vi "Remove Lens Distortion.vi"(2 "error in (no error)":errorcluster, 3 "Image Dst":T1, 4 "Calibration Image":T1) -> (0 "error out":errorcluster, 1 "Corrected Image":T1)   [LabVIEW 2009, in "Camera.lvlib" / "Lens Distortion.lvlib"]
doc: "Removes lens distortion in a image using a calibration image"
uses:
  <vilib>/vision/Image Controls.llb/IMAQ Image.ctl
  Lens Distortion.lvlib
  <vilib>/vision/NI_Vision_Development_Module.lvlib
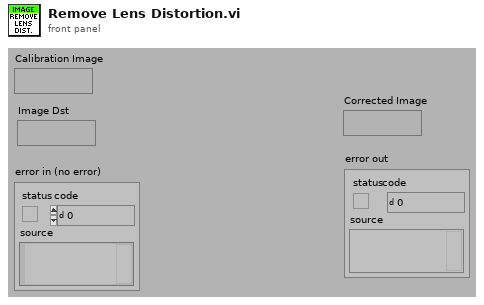
[diagram p1: front panel]
types:
  T1 = typedef "IMAQ Image.ctl" = refnum<image>
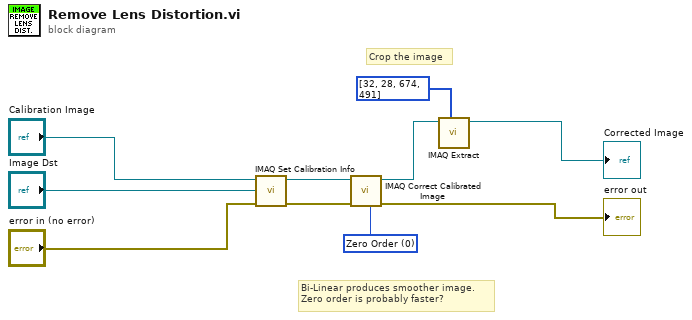
[diagram p0: block diagram]
diagram:
  w10 = u32 0 items=["Zero Order", "Bi-Linear", "Quadratic", "Cubic Spline"] ("Interpolation Type")
  # "Crop the image"
  # "Bi-Linear produces smoother image.\nZero order is probably faster?"
  n1 = call "IMAQ Set Calibration Info"("error in (no error)"="error in (no error)", "Image Dst"="Image Dst", "Image Src"="Calibration Image") -> ("error out"=w5:errorcluster, "Calibrated Image"=w9:T1)  [unwired: 1 in, 6 out]
  n2 = call "IMAQ Correct Calibrated Image"("Interpolation Type"=w10, "error in (no error)"=w5, "Image Src"=w9) -> ("error out"=→"error out":errorcluster, "Corrected Image"=w2:T1)  [unwired: 7 in]
  n3 = call "IMAQ Extract"("Optional Rectangle"=i32[] [32, 28, 674, 491], "Image Src"=w2) -> ("Image Dst Out"=→"Corrected Image":T1)  [unwired: 8 in, 1 out]
